vi "Acoustic Calibration.vi"(0 "TSM context":T1, 5 "Cal File Path":path) -> (15 "error out":errorcluster)   [LabVIEW 2020]
doc: "Generates a Acoustic Calibration File with calibration data of each Site. Acoustic calibration for the DUT is obtained by sweeping over Amplitude and Frequency logarithmically and finding out the respective dB SPL. Then with the obtained dB SPL, Frequency and Amplitude information for each site is logged into calibration file along with other information's like TEDS, Site number and serial number."
uses:
  <vilib>/NI_TestStand_SemiconductorModule/NI_TestStand_Semiconductor_Module.lvlibp/PinMap/General/SemiconductorModuleContext.ctl
  Common/Utility/Calibration Sweep/Sweep Parameters.ctl
  Common/Utility/Calibration File API/Acoustic Cal Data Cluster.ctl
  <vilib>/NI_TestStand_SemiconductorModule/NI_TestStand_Semiconductor_Module.lvlibp
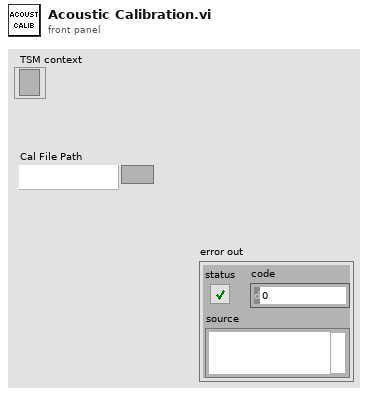
[diagram p1: front panel]
types:
  T1 = typedef "NI_TestStand_Semiconductor_Module.lvlibp/SemiconductorModuleContext.ctl" = refnum<k7>
  T2 = typedef "Sweep Parameters.ctl" = cluster{"Start":dbl, "End":dbl, "Samples":i32}
  T3 = typedef "Acoustic Cal Data Cluster.ctl" = cluster{"Site Number":i32, "Serial Number":u32, "Ref Mic Sensitivity":dbl, "SPL Axis":dbl[], "Frequency Axis":dbl[], "Speaker Vp":dbl[][], "Ref Mic Cal File Data":string[][], "Speaker Vp Axis":dbl[], "SPL Measurements":dbl[][]}
  T4 = cluster{"TSM context":T1, "Site Numbers":i32[], "Ref Mic Sampling Rate (Hz)":dbl, "Speaker Sampling Rate (Hz)":dbl, "Cal File Path":path, "Coarse Frequency Sweep":T2, "Fine Frequency Sweep":T2, "Coarse Amplitude Sweep":T2, "Fine Amplitude Sweep":T2, "Frequency Sweep (Hz)":dbl[], "Amplitude Sweep (V)":dbl[], "Per-Site Per-Freq Per-Amp dB SPL":dbl[][][], "Acoustic Cal Data":T3[], "Start dB SPL":dbl, "End dB SPL":dbl, "dB SPL Increment":dbl}
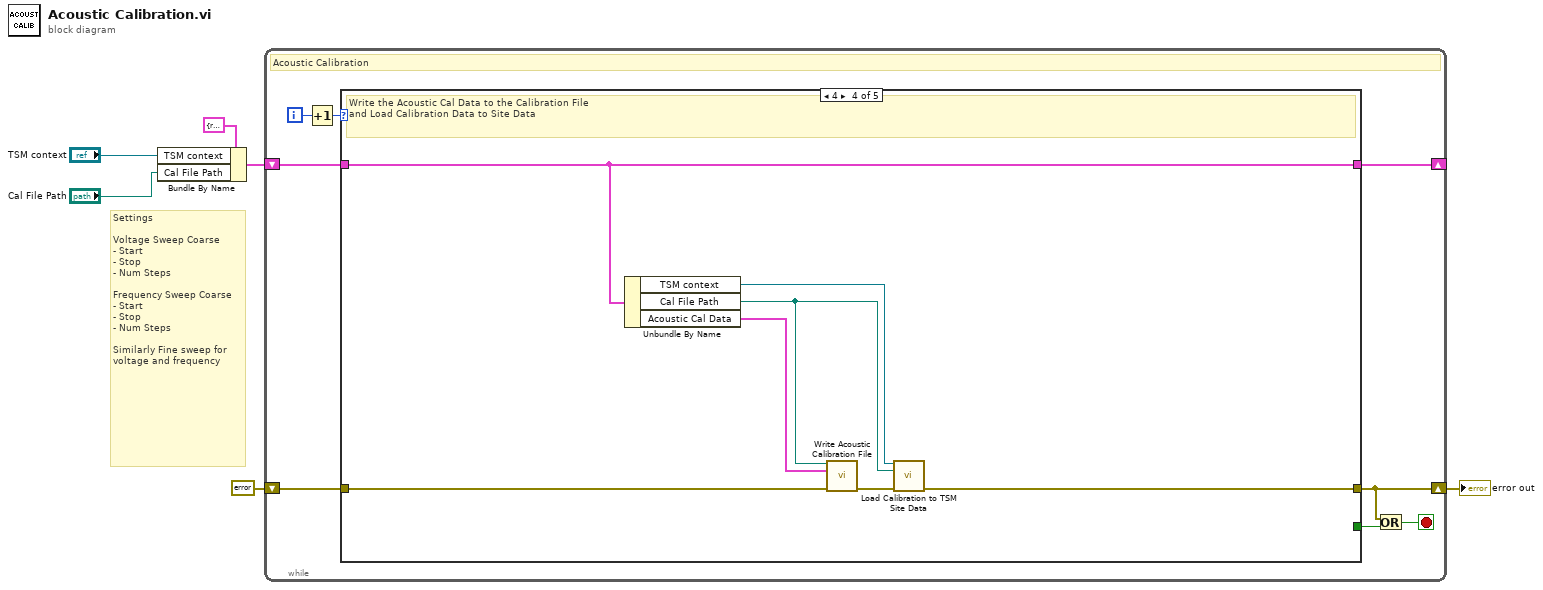
[diagram p0: block diagram]
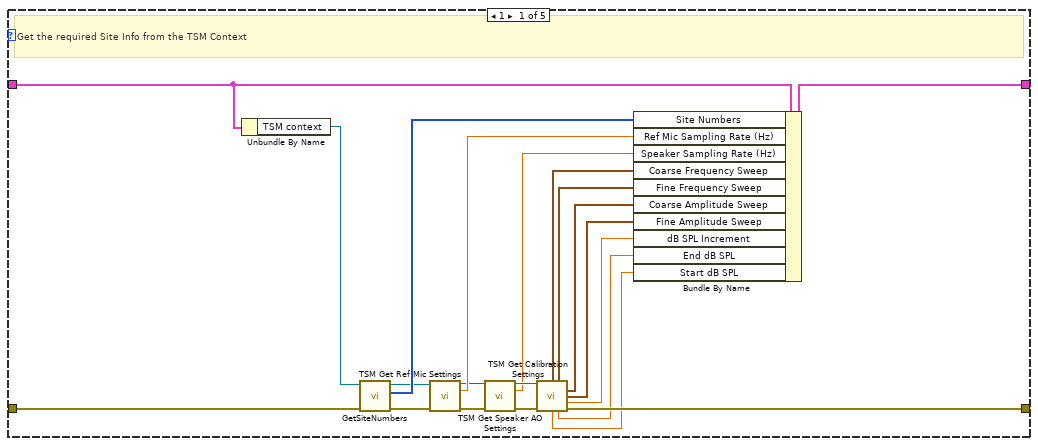
[diagram p2: hidden frame]
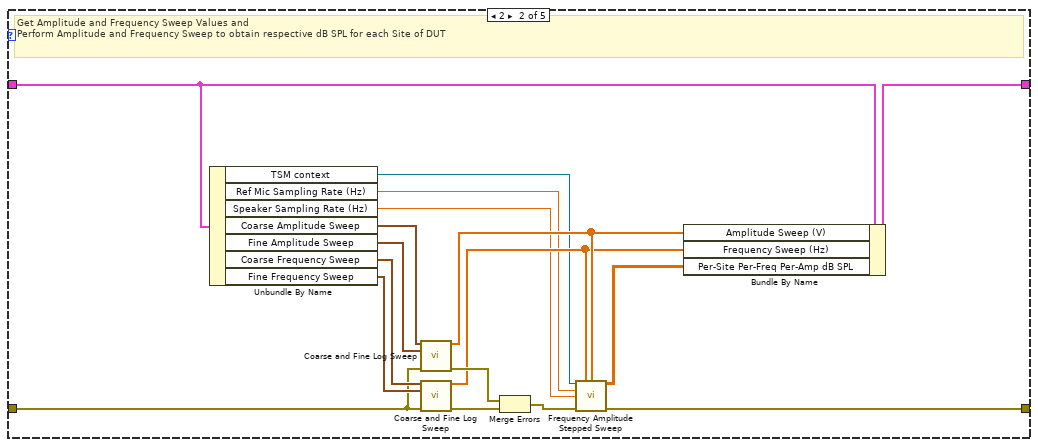
[diagram p3: hidden frame]
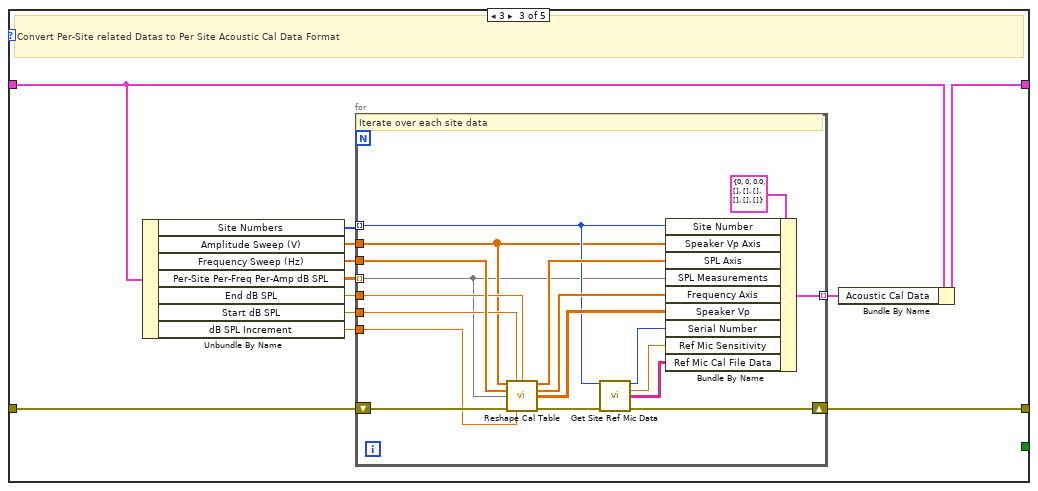
[diagram p4: hidden frame]
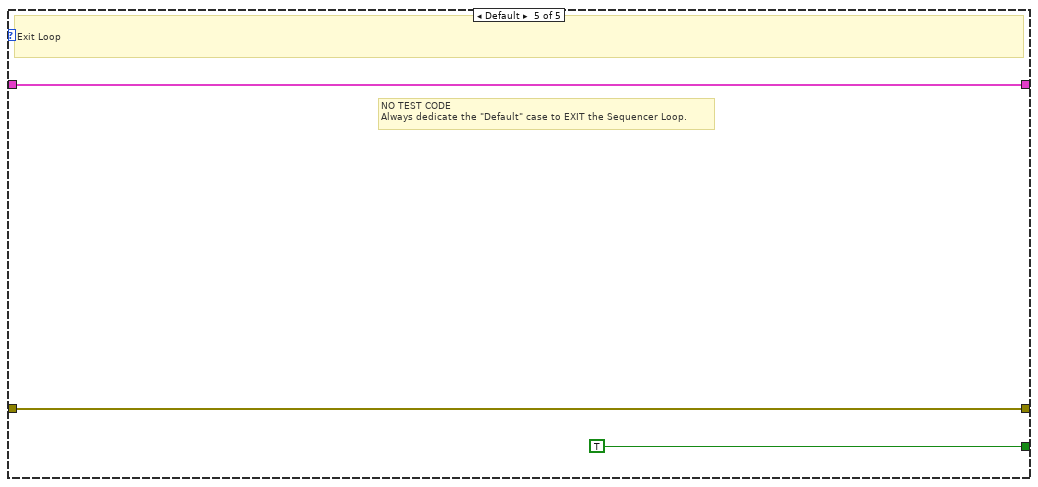
[diagram p5: hidden frame]
diagram:
  # "Settings\n\nVoltage Sweep Coarse\n- Start\n- Stop\n- Num Steps\n\nFrequency Sweep Coarse\n- Start\n- Stop\n- Num Steps\n\nSimilarly Fine sweep for \nvoltage and frequency"
  n1 = Bundle By Name(cluster=T4 {"TSM context"=refnum, "Site Numbers"=[], "Ref Mic Sampling Rate (Hz)"=0.0, "Speaker Sampling Rate (Hz)"=0.0, "Cal File Path"=path "", "Coarse Frequency Sweep"={"Start"=20.0, "End"=20000.0, "Samples"=128}, "Fine Frequency Sweep"={"Start"=20.0, "End"=20000.0, "Samples"=128}, "Coarse Amplitude Sweep"={"Start"=20.0, "End"=20000.0, "Samples"=128}, "Fine Amplitude Sweep"={"Start"=20.0, "End"=20000.0, "Samples"=128}, "Frequency Sweep (Hz)"=[], "Amplitude Sweep (V)"=[], "Per-Site Per-Freq Per-Amp dB SPL"=[], "Acoustic Cal Data"=[], "Start dB SPL"=0.0, "End dB SPL"=0.0, "dB SPL Increment"=0.0}, "TSM context"="TSM context", "Cal File Path"="Cal File Path") -> (w1:T4)
  n2 = while {
    shift-right: [w7] -> w6
    shift-left: errorcluster {"status"=FALSE, "code"=0, "source"=""} ("error in") -> [w13]
    shift-right: [w10] -> _
    shift-left: w1 -> [w11]
    i -> [w14]
    stop <- w8 stop-if-true
    # "Acoustic Calibration"
    n3 = Increment(x=w14) -> (x+1=w12:i32)
    n4 = case shown="4" w12 {
      tunnel: [w27 w43 w61 w85 w92] -> w7
      tunnel: w13 -> [w35 w36 w62 w89 w92]
      tunnel: w11 -> [w32 w52 w64 w88 w91]
      tunnel: [w34 w51 w60 w88 w91] -> w10
      tunnel: [_ _ _ _ TRUE] -> w9
      frame 1 {
        # "Get the required Site Info from the TSM Context"
        n5 = Unbundle By Name(w32) -> ("TSM context"=w31:T1)
        n6 = call <vilib>:"GetSiteNumbers.vi"("error in (no error)"=w35, "Semiconductor Module Context"=w31) -> ("error out"=w30:errorcluster, "Site Numbers"=w33:i32[], "Semiconductor Module Context Out"=w29:T1)  [unwired: 6 in, 1 out]
        n7 = call "TSM Get Ref Mic Settings.vi"("TSM context"=w29, "error in (no error)"=w30) -> ("TSM context Out"=w17:T1, "Sampling Rate (Hz)"=w28:dbl, "error out"=w19:errorcluster)  [unwired: 8 in, 3 out]
        n8 = call "TSM Get Speaker AO Settings.vi"("TSM context"=w17, "error in (no error)"=w19) -> ("TSM context Out"=w16:T1, "Sampling Rate (Hz)"=w15:dbl, "error out"=w18:errorcluster)  [unwired: 9 in, 2 out]
        n9 = call "TSM Get Calibration Settings.vi"("TSM context"=w16, "error in (no error)"=w18) -> ("Coarse Freq Sweep (Hz)"=w20:T2, "Fine Freq Sweep (Hz)"=w26:T2, "Coarse Amp Sweep (Hz)"=w25:T2, "Fine Amp Sweep (Hz)"=w24:T2, "dB SPL Increment"=w23:dbl, "Start dB SPL"=w21:dbl, "End dB SPL"=w22:dbl, "error out"=w27:errorcluster)  [unwired: 5 in, 1 out]
        n10 = Bundle By Name(cluster=w32, "Site Numbers"=w33, "Ref Mic Sampling Rate (Hz)"=w28, "Speaker Sampling Rate (Hz)"=w15, "Coarse Frequency Sweep"=w20, "Fine Frequency Sweep"=w26, "Coarse Amplitude Sweep"=w25, "Fine Amplitude Sweep"=w24, "dB SPL Increment"=w23, "End dB SPL"=w22, "Start dB SPL"=w21) -> (w34:T4)
      }
      frame 2 {
        # "Get Amplitude and Frequency Sweep Values and\nPerform Amplitude and Frequency Sweep to obtain respective dB SPL for each Site of DUT"
        n11 = Unbundle By Name(w52) -> ("TSM context"=w41:T1, "Ref Mic Sampling Rate (Hz)"=w40:dbl, "Speaker Sampling Rate (Hz)"=w37:dbl, "Coarse Amplitude Sweep"=w38:T2, "Fine Amplitude Sweep"=w48:T2, "Coarse Frequency Sweep"=w50:T2, "Fine Frequency Sweep"=w49:T2)
        n12 = call "Coarse and Fine Log Sweep.vi"("Coarse Sweep"=w38, "Fine Sweep"=w48, "error in (no error)"=w36) -> ("Sweep Values"=w47:dbl[], "error out"=w45:errorcluster)  [unwired: 11 in]
        n13 = call "Coarse and Fine Log Sweep.vi"("Coarse Sweep"=w50, "Fine Sweep"=w49, "error in (no error)"=w36) -> ("Sweep Values"=w42:dbl[], "error out"=w46:errorcluster)  [unwired: 11 in]
        n14 = Merge Errors(w45, w46) -> (w44:errorcluster)
        n15 = call "Frequency Amplitude Stepped Sweep.vi"("Semiconductor Module Context"=w41, "Frequency Sweep (Hz)"=w42, "Amplitude Sweep (V)"=w47, "Ref Mic Sampling Rate (Hz)"=w40, "Speaker Sampling Rate (Hz)"=w37, "error in (no error)"=w44) -> ("Per-Site Per-Freq Per-Amp dB SPL"=w39:dbl[][][], "error out"=w43:errorcluster)  [unwired: 8 in]
        n16 = Bundle By Name(cluster=w52, "Amplitude Sweep (V)"=w47, "Frequency Sweep (Hz)"=w42, "Per-Site Per-Freq Per-Amp dB SPL"=w39) -> (w51:T4)
      }
      frame 3 {
        # "Convert Per-Site related Datas to Per Site Acoustic Cal Data Format"
        n17 = Unbundle By Name(w64) -> ("Site Numbers"=w56:i32[], "Amplitude Sweep (V)"=w58:dbl[], "Frequency Sweep (Hz)"=w57:dbl[], "Per-Site Per-Freq Per-Amp dB SPL"=w63:dbl[][][], "End dB SPL"=w55:dbl, "Start dB SPL"=w54:dbl, "dB SPL Increment"=w53:dbl)
        n18 = for {
          tunnel: [w78] -> w59 mode=indexing
          tunnel: w63 -> [w65] mode=indexing
          shift-right: [w70] -> w61
          shift-left: w62 -> [w76]
          tunnel: w58 -> [w66]
          tunnel: w57 -> [w77]
          tunnel: w56 -> [w71] mode=indexing
          tunnel: w55 -> [w75]
          tunnel: w54 -> [w74]
          tunnel: w53 -> [w73]
          # "Iterate over each site data"
          n19 = call "Reshape Cal Table.vi"("Speaker amplitudes"=w66, "Start dB SPL"=w74, "End dB SPL"=w75, "Frequencies"=w77, "Measured dB SPL"=w65, "error in (no error)"=w76, "dB SPL Increment"=w73) -> ("dB SPL Axis"=w81:dbl[], "Frequency Axis"=w80:dbl[], "Speaker amplitude"=w79:dbl[][], "error out"=w72:errorcluster)  [unwired: 5 in]
          n20 = call "Get Site Ref Mic Data.vi"("Site Number"=w71, "error in (no error)"=w72) -> ("Serial Number"=w69:u32, "Ref Mic Sensitivity (mV/Pa)"=w68:dbl, "Ref Mic Cal File Data"=w67:string[][], "error out"=w70:errorcluster)  [unwired: 10 in]
          n21 = Bundle By Name(cluster=T3 {"Site Number"=0, "Serial Number"=0, "Ref Mic Sensitivity"=0.0, "SPL Axis"=[], "Frequency Axis"=[], "Speaker Vp"=[], "Ref Mic Cal File Data"=[], "Speaker Vp Axis"=[], "SPL Measurements"=[]} ("Acoustic Cal Data"), "Site Number"=w71, "Speaker Vp Axis"=w66, "SPL Axis"=w81, "SPL Measurements"=w65, "Frequency Axis"=w80, "Speaker Vp"=w79, "Serial Number"=w69, "Ref Mic Sensitivity"=w68, "Ref Mic Cal File Data"=w67) -> (w78:T3)
        }
        n22 = Bundle By Name(cluster=w64, "Acoustic Cal Data"=w59) -> (w60:T4)
      }
      frame 4 {
        # "Write the Acoustic Cal Data to the Calibration File\nand Load Calibration Data to Site Data"
        n23 = Unbundle By Name(w88) -> ("TSM context"=w84:T1, "Cal File Path"=w83:path, "Acoustic Cal Data"=w87:T3[])
        n24 = call "Write Acoustic Calibration File.vi"("Cal File Path"=w83, "Per Site Acoustic Cal Data"=w87, "error in (no error)"=w89) -> ("error out"=w86:errorcluster)  [unwired: 12 in]
        n25 = call "Load Calibration to TSM Site Data.vi"("TSM context"=w84, "Cal File Path"=w83, "error in"=w86) -> ("error out"=w85:errorcluster)  [unwired: 12 in]
      }
      frame Default {
        (unwired) TRUE
        # "NO TEST CODE\nAlways dedicate the \"Default\" case to EXIT the Sequencer Loop."
        # "Exit Loop"
      }
    }
    n26 = Or(x=w7, y=w9) -> (x .or. y?=w8:bool)
  }
  "error out" <- w6
